vi "Close MB.vi"(8 "error in (no error)":errorcluster, 11 "DAM0404D in":refnum<class "DAM0404D.lvclass">) -> (0 "error out":errorcluster, 3 "DAM0404D out":refnum<class "DAM0404D.lvclass">)   [LabVIEW 2016, in "DAM0404D.lvlib" / "DAM0404D.lvclass"]
uses:
  DAM0404D.lvclass
  DAM0404D.lvclass/DAM0404D.ctl
  <vilib>/Plasmionique/MB Master/MB_Master/MB_Master.lvclass
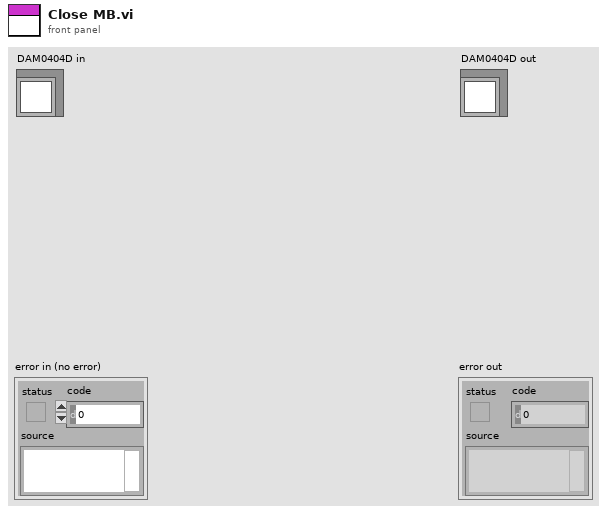
[diagram p1: front panel]
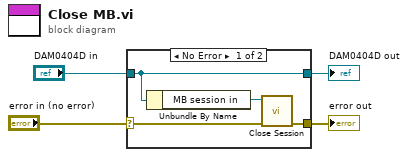
[diagram p0: block diagram]
diagram:
  n1 = case shown="No Error" "error in (no error)" {
    selector: "error in (no error)" -> [w5 w10]
    tunnel: [w6 w10] -> w3
    tunnel: [w8 w9] -> w1
    tunnel: "DAM0404D in" -> [w8 w9]
    frame No Error {
      n2 = Unbundle By Name(w8) -> ("MB session in"=w7:refnum<class "MB_Master.lvclass">)
      n3 = call-dynamic "Close Session.vi"("error in (no error)"=w5, "MB session in"=w7) -> ("error out"=w6:errorcluster)  [unwired: 9 in]
    }
    frame Error {
    }
  }
  "error out" <- w3
  "DAM0404D out" <- w1
